vi "Create Channel.vi"(6 "index":i32, 8 "error in":errorcluster, 10 "channel settings":T1, 11 "counter driven output mode in":refnum<class "Counter Driven Output Mode.lvclass">) -> (0 "error out":errorcluster, 2 "counter driven output channel":refnum<class "Counter Driven Output Channel.lvclass">, 3 "counter driven output mode out":refnum<class "Counter Driven Output Mode.lvclass">)   [LabVIEW 2020, in "Scan Engine Scripting.lvlib" / "Counter Driven Output Mode.lvclass"]
uses:
  Counter Driven Output Mode.lvclass
  Controls/counter driven output channel settings.ctl
  Channel Classes/Counter Driven Output Channel/Counter Driven State.ctl
  Channel Classes/Counter Driven Output Channel/Counter Driven Output Channel.lvclass
  Counter Driven Output Mode.lvclass/Counter Driven Output Mode.ctl
  Scan Engine Scripting.lvlib
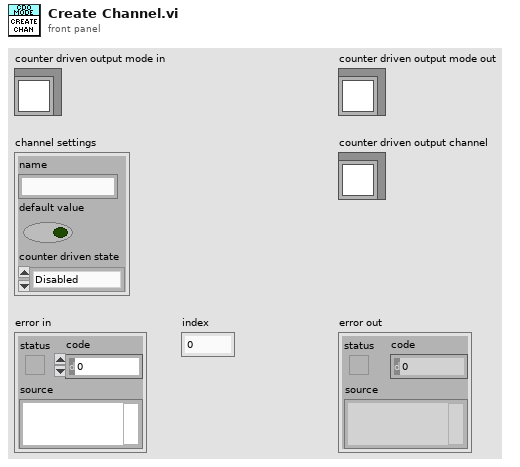
[diagram p1: front panel]
types:
  T1 = typedef "Scan Engine Scripting.lvlib/counter driven output channel settings.ctl" = cluster{"name":string, "default value":bool, "counter driven state":T2}
  T2 = typedef "Scan Engine Scripting.lvlib/Counter Driven Output Channel.lvclass/Counter Driven State.ctl" = enum16{"Disabled", "Enabled"}
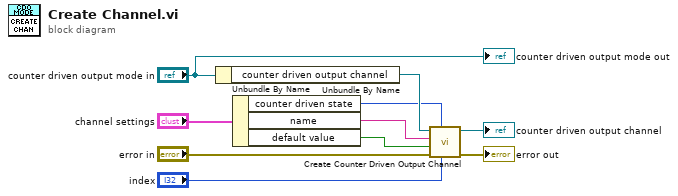
[diagram p0: block diagram]
diagram:
  n1 = Unbundle By Name("counter driven output mode in") -> ("counter driven output channel"=w4:refnum<class "Counter Driven Output Channel.lvclass">)
  n2 = Unbundle By Name("channel settings") -> ("counter driven state"=w1:T2, "name"=w3:string, "default value"=w2:bool)
  n3 = call-dynamic "Create Counter Driven Output Channel.vi"("index"="index", "counter driven state"=w1, "error in"="error in", "default value"=w2, "name"=w3, "counter driven output channel in"=w4) -> ("error out"=→"error out":errorcluster, "counter driven output channel out"=→"counter driven output channel":refnum<class "Counter Driven Output Channel.lvclass">)  [unwired: 4 in]
  "counter driven output mode out" <- "counter driven output mode in"
